vi "Write Initialized.vi"(8 "error in (no error)":errorcluster, 10 "Initialized":bool, 11 "MB Slave Simulator Base in":refnum<class "MB Slave Simulator Base.lvclass">) -> (0 "error out":errorcluster, 3 "MB Slave Simulator Base out":refnum<class "MB Slave Simulator Base.lvclass">)   [LabVIEW 2021, in "MB Slave Simulator Base.lvclass"]
uses:
  MB Slave Simulator Base.lvclass
  MB Slave Simulator Base.lvclass/MB Slave Simulator Base.ctl
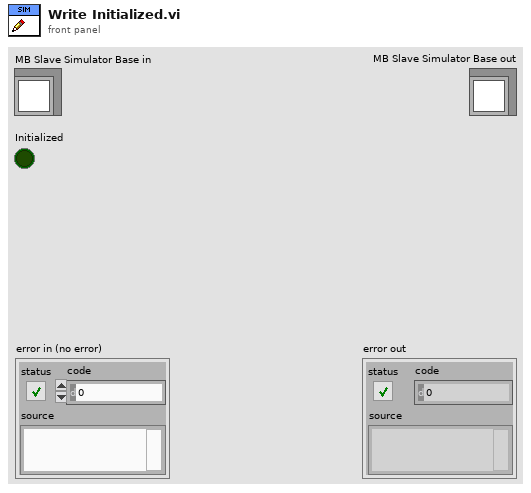
[diagram p1: front panel]
types:
  T1 = typedef "MB Slave Simulator Base.lvclass/dvr_type.ctl" = cluster{"_PARMS":T2, "state_vars":T5}
  T2 = typedef "MB Slave Simulator Base.lvclass/_PARMS.ctl" = cluster{"ch_alias":string[], "ch_units":string[], "Modules to Launch":T3[]}
  T3 = typedef "Module.lvclass/Launch Module Typdef.ctl" = cluster{"Module":string, "Parameters":T4}
  T4 = typedef "Module.lvclass/Launch Module Parms.ctl" = cluster{"Name":string, "Arguments":string[], "Show FP?":bool}
  T5 = typedef "MB Slave Simulator Base.lvclass/state_vars.ctl" = cluster{"Initialized":bool}
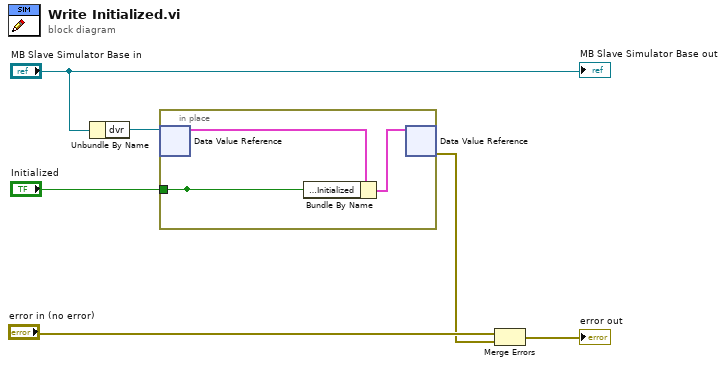
[diagram p0: block diagram]
diagram:
  n1 = Unbundle By Name ("DVR Unbundle")("MB Slave Simulator Base in") -> ("dvr"=w2:refnum<data-value>)
  n2 = in-place "In Place Element Structure" {
    in-place-border: [w7] -> _
    in-place-border: "Initialized" -> [w7]
    n3 = in-place-dvr #1(w2) -> (w9:T1)  [unwired: 1 out]
    n4 = Bundle By Name ("Item Bundle")(cluster=w9, "state_vars.Initialized"=w7) -> (w8:T1)
    n5 = in-place-dvr #1(w8) -> (w3:errorcluster)  [unwired: 1 out]
  }
  n6 = Merge Errors("error in (no error)", w3) -> (→"error out":errorcluster)
  "MB Slave Simulator Base out" <- "MB Slave Simulator Base in"
